vi "Toolkit Post-Install Custom Action.vi"(10 "Variant":variant) -> (0 "error out":errorcluster)   [LabVIEW 2020]
uses:
  <vilib>/Utility/traverseref.llb/TRef TravTarget.ctl
  <vilib>/Utility/traverseref.llb/VI Scripting - Traverse.lvlib
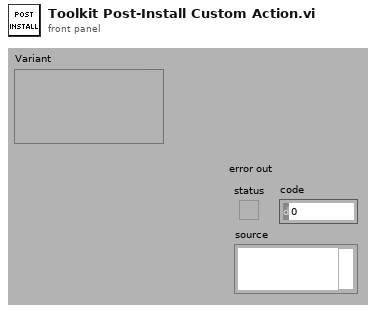
[diagram p1: front panel]
types:
  T1 = typedef "TRef TravTarget.ctl" = enum16{"FP", "BD", "Other"}
  T2 = typedef "LVPositionTypeDef.ctl" = cluster{"Left":i32, "Top":i32}
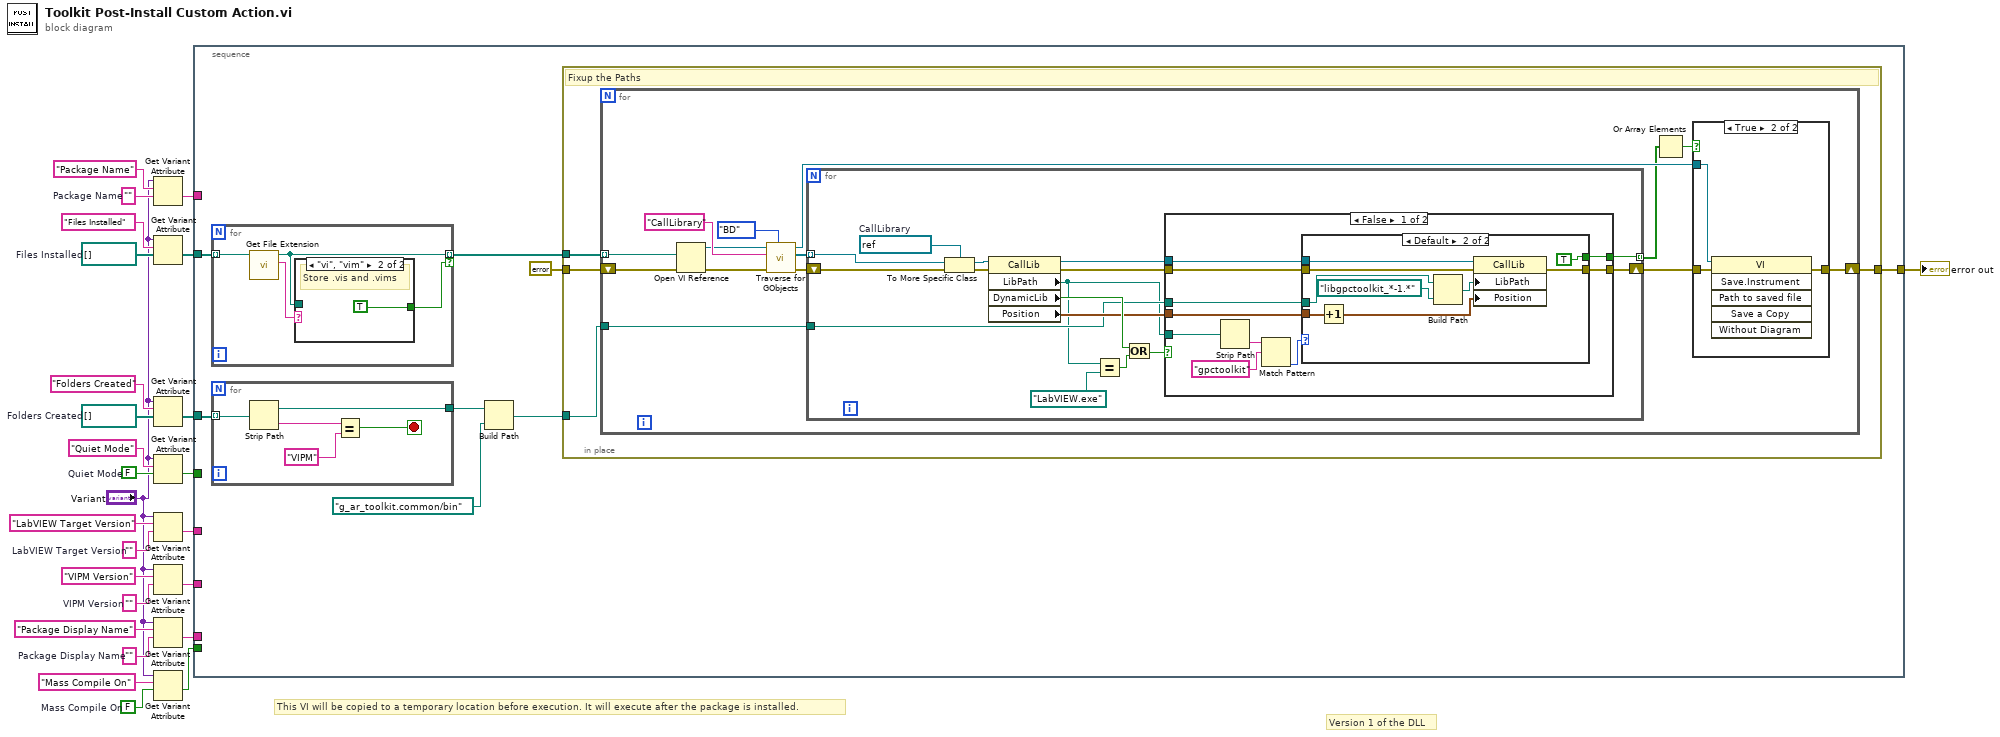
[diagram p0: block diagram]
diagram:
  w3 = path[] []  # Folders Created
  w4 = path[] []  # Files Installed
  w9 = FALSE  # Mass Compile On
  w10 = ""  # Package Display Name
  w17 = FALSE  # Quiet Mode
  w20 = ""  # VIPM Version
  w22 = ""  # LabVIEW Target Version
  w24 = ""  # Package Name
  # "Version 1 of the DLL"
  # "This VI will be copied to a temporary location before execution. It will execute after the package is installed."
  n1 = Get Variant Attribute(Variant="Variant", name="Package Name", default value (empty Variant)=w24) -> (value=w15:string)  [unwired: 1 in, 3 out]
  n2 = Get Variant Attribute(Variant="Variant", name="Files Installed", default value (empty Variant)=w4) -> (value=w6:path[])  [unwired: 1 in, 3 out]
  n3 = Get Variant Attribute(Variant="Variant", name="Folders Created", default value (empty Variant)=w3) -> (value=w7:path[])  [unwired: 1 in, 3 out]
  n4 = Get Variant Attribute(Variant="Variant", name="Quiet Mode", default value (empty Variant)=w17) -> (value=w12:bool)  [unwired: 1 in, 3 out]
  n5 = Get Variant Attribute(Variant="Variant", name="LabVIEW Target Version", default value (empty Variant)=w22) -> (value=w14:string)  [unwired: 1 in, 3 out]
  n6 = Get Variant Attribute(Variant="Variant", name="VIPM Version", default value (empty Variant)=w20) -> (value=w13:string)  [unwired: 1 in, 3 out]
  n7 = Get Variant Attribute(Variant="Variant", name="Package Display Name", default value (empty Variant)=w10) -> (value=w16:string)  [unwired: 1 in, 3 out]
  n8 = Get Variant Attribute(Variant="Variant", name="Mass Compile On", default value (empty Variant)=w9) -> (value=w11:bool)  [unwired: 1 in, 3 out]
  n9 = stacked-sequence {
    tunnel: w16 -> [_]
    tunnel: w15 -> [_]
    tunnel: w14 -> [_]
    tunnel: w13 -> [_]
    tunnel: w12 -> [_]
    tunnel: w11 -> [_]
    tunnel: w6 -> [w34]
    tunnel: w7 -> [w33]
    tunnel: [w29] -> w2
    frame #0 {
      n10 = for {
        tunnel: w34 -> [w43] mode=indexing
        tunnel: [w40] -> w32 mode=indexing if=w41
        n11 = call <vilib>:"Get File Extension.vi"("file"=w43) -> ("lowercase file extension"=w42:string, "dup file"=w40:path)  [unwired: 6 in, 3 out]
        n12 = case shown="\"vi\", \"vim\"" w42 {
          tunnel: [_ TRUE] -> w41
          tunnel: w40 -> [_ _]
          frame Default {
          }
          frame "vi", "vim" {
            # "Store .vis and .vims"
          }
        }
      }
      n13 = for {
        tunnel: w33 -> [w39] mode=indexing
        tunnel: [w38] -> w28
        stop <- w36 stop-if-true
        n14 = Strip Path(path=w39) -> (stripped path=w38:path, name=w37:string)
        n15 = Equal?(x=w37, y="VIPM") -> (x = y?=w36:bool)
      }
      n16 = Build Path(base path=w28, name or relative path=path "g_ar_toolkit.common/bin") -> (appended path=w30:path)
      n17 = in-place {
        in-place-border: [w46] -> w29
        in-place-border: w32 -> [w48]
        in-place-border: errorcluster {"status"=FALSE, "code"=0, "source"=""} ("error in (no error)") -> [w47]
        in-place-border: w30 -> [w45]
        # "Fixup the Paths"
        n18 = for {
          tunnel: w48 -> [w60] mode=indexing
          shift-right: [w58] -> w46
          shift-left: w47 -> [w57]
          tunnel: w45 -> [w49]
          n19 = Open VI Reference(vi path=w60, error in (no error)=w57) -> (vi reference=w53:refnum<vi>, error out=w52:errorcluster)  [unwired: 4 in]
          n20 = call <vilib>:"Traverse for GObjects.vi"("Traverse Target"=TRef_TravTarget."BD", "error in (no error)"=w52, "Class Name"="CallLibrary", "VI Refnum"=w53) -> ("error out"=w56:errorcluster, "References"=w51:refnum<vi>[], "dup VI Refnum"=w62:refnum<vi>)  [unwired: 4 in, 1 out]
          n21 = for {
            tunnel: w51 -> [w71] mode=indexing
            shift-right: [w78] -> w61
            shift-left: w56 -> [w73]
            tunnel: [w69] -> w50 mode=indexing
            tunnel: w49 -> [w67]
            w72 = refnum<vi> refnum  # CallLibrary
            n22 = To More Specific Class(target class=w72, reference=w71, error in=w73) -> (specific class reference=w74:refnum<vi>, error out=w75:errorcluster)
            n23 = property class="CallLib"(reference=w74, error in=w75) -> (reference out=w77:refnum<vi>, error out=w76:errorcluster, "LibPath"=w64:path, "DynamicLib"=w70:bool, "Position"=w68:T2)
            n24 = Equal?(x=w64, y=path "LabVIEW.exe") -> (x = y?=w65:bool)
            n25 = Or(x=w70, y=w65) -> (x .or. y?=w66:bool)
            n26 = case shown="False" w66 {
              tunnel: [w88 w99] -> w78
              tunnel: w77 -> [w87 _]
              tunnel: w76 -> [w86 w99]
              tunnel: w64 -> [w83 _]
              tunnel: [w82 _] -> w69
              tunnel: w68 -> [w80 _]
              tunnel: w67 -> [w79 _]
              frame False {
                n27 = Strip Path(path=w83) -> (name=w84:string)  [unwired: 1 out]
                n28 = Match Pattern(string=w84, regular expression="gpctoolkit") -> (offset past match=w81:i32)  [unwired: 1 in, 3 out]
                n29 = case shown="Default" w81 {
                  tunnel: [w89 w98] -> w88
                  tunnel: w87 -> [_ w96]
                  tunnel: w86 -> [w89 w95]
                  tunnel: [_ TRUE] -> w82
                  tunnel: w80 -> [_ w92]
                  tunnel: w79 -> [_ w90]
                  frame -1 {
                  }
                  frame Default {
                    n30 = Increment(x=w92) -> (x+1=w93:T2)
                    n31 = Build Path(base path=w90, name or relative path=path "libgpctoolkit_*-1.*") -> (appended path=w97:path)
                    n32 = property class="CallLib"(reference=w96, error in=w95, "LibPath"=w97, "Position"=w93) -> (error out=w98:errorcluster)  [unwired: 1 out]
                  }
                }
              }
              frame True {
              }
            }
          }
          n33 = Or Array Elements(Boolean array=w50) -> (logical OR=w59:bool)
          n34 = case shown="True" w59 {
            tunnel: w62 -> [_ w102]
            tunnel: w61 -> [w100 w101]
            tunnel: [w100 w103] -> w58
            frame False {
            }
            frame True {
              n35 = invoke class="VI" method="Save.Instrument"(reference=w102, error in=w101) -> (error out=w103:errorcluster)  [unwired: 4 in, 5 out]
            }
          }
        }
      }
    }
  }
  "error out" <- w2
